vi "游标.vi"() -> ()   [LabVIEW 2010]
uses:
  <vilib>/Analysis/NI_AALBase.lvlib
panel:
  out "波形图":dbl[][](graph)
  # "⑴    ⑵                     ⑶       ⑷                                ⑸"
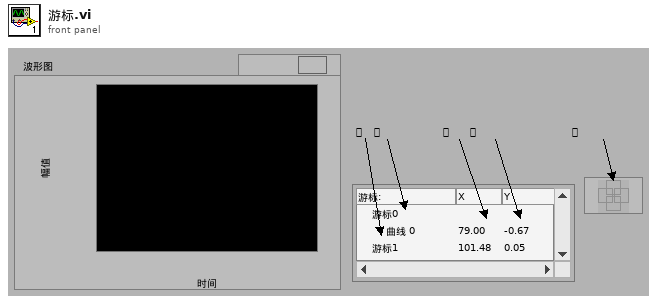
[diagram p1: front panel]
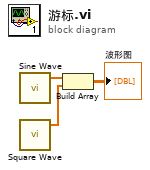
[diagram p0: block diagram]
diagram:
  n1 = call <vilib>:"Sine Wave.vi"() -> ("sine wave"=w2:dbl[])  [unwired: 5 in, 2 out]
  n2 = call <vilib>:"Square Wave.vi"() -> ("square wave"=w1:dbl[])  [unwired: 6 in, 2 out]
  n3 = Build Array(w2, w1) -> (→"波形图":dbl[][])
